vi "浮点数正则表达式（任意精度，单词）.vi"(8 "error in (no error)":errorcluster caption="错误输入（无错误）") -> (0 "error out":errorcluster caption="错误输出", 3 "正则表达式":string)   [LabVIEW 2011]
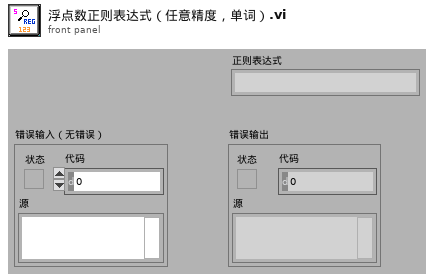
[diagram p1: front panel]
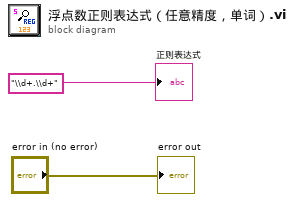
[diagram p0: block diagram]
diagram:
  "正则表达式" <- "\\d+.\\d+" ("格式字符串")
  "error out" <- "error in (no error)"
